vi "YKMW100 Get Com Log.vi"(0 "VISA session":refnum<visa-resource-name>="MW100", 2 "Semiphore":T1, 9 "Timeout (25000)":u32=100, 11 "error in (no error)":errorcluster, 13 "Source (\"\")":string) -> (4 "dup VISA session":refnum<visa-resource-name>, 6 "Com History":string[](array[string]), 7 "Send Message (\"\")":string, 15 "error out":errorcluster)   [LabVIEW 2009]
doc: "This VI sends the message. Then it returns the response."
panel:
  out "Read Buffer":string
  in  "Number of Read Blocks (1-200)":i32=200
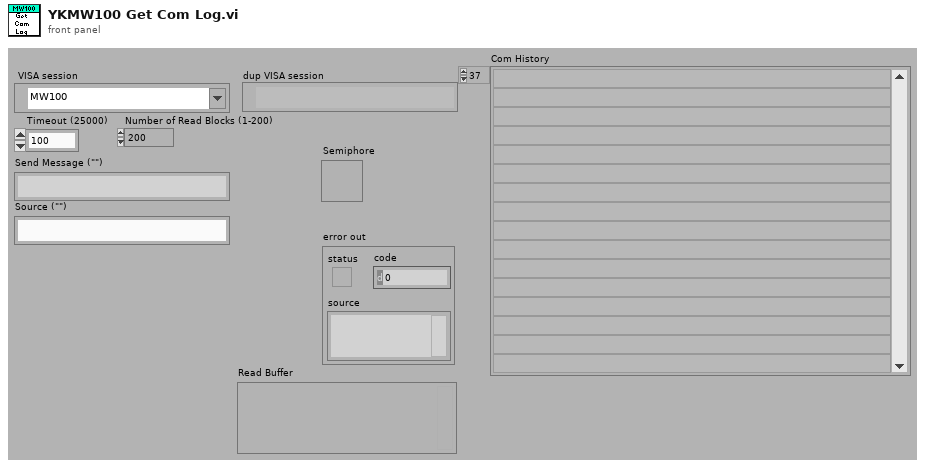
[diagram p1: front panel]
types:
  T1 = typedef "Semaphore RefNum" = refnum<k1>
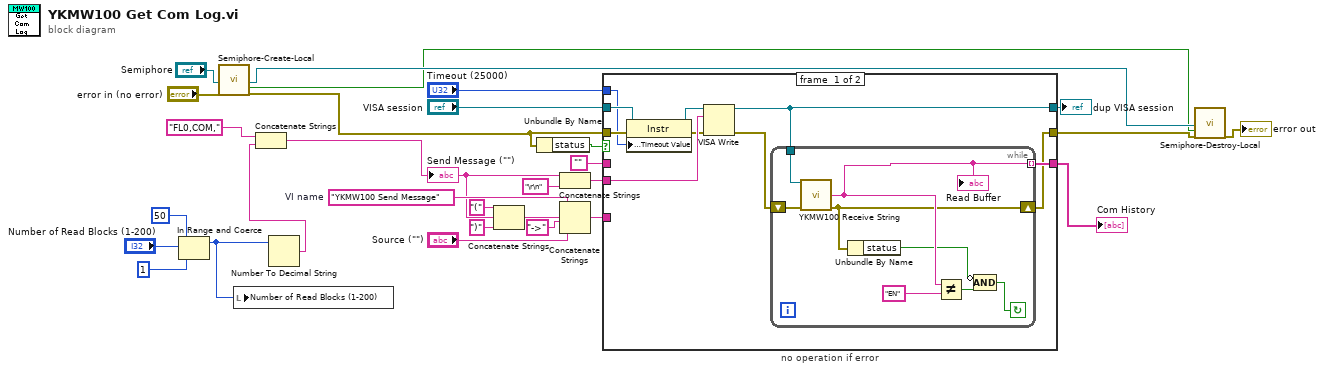
[diagram p0: block diagram]
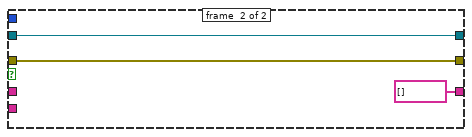
[diagram p2: hidden frame]
diagram:
  w19 = "YKMW100 Send Message"  # VI name
  n1 = In Range and Coerce(upper limit=50, x="Number of Read Blocks (1-200)", lower limit=1) -> (coerced(x)=w11:i32)  [unwired: 1 out]
  n2 = call "Semiphore-Create-Local.vi"("Semiphore"="Semiphore", "error in (no error)"="error in (no error)") -> ("semaphore"=w2:T1, "Local?"=w1:bool, "error out"=w5:errorcluster)  [unwired: 15 in]
  n3 = local write "Number of Read Blocks (1-200)"(w11) -> ()
  n4 = Number To Decimal String(number=w11) -> (decimal integer string=w10:string)  [unwired: 1 in]
  n5 = Concatenate Strings("FL0,COM,", w10) -> (w9:string)
  "Send Message (\"\")" <- w9
  n6 = Concatenate Strings("(", w9, ")") -> (w20:string)
  n7 = Unbundle By Name(w5) -> ("status"=w26:bool)
  n8 = Concatenate Strings(w9, "\r\n") -> (w29:string)
  n9 = Concatenate Strings(w19, w20, "->", "Source (\"\")") -> (w25:string)
  n10 = case "no operation if error" shown="False" w26 {
    tunnel: "VISA session" -> [w36 w50]
    tunnel: w29 -> [w39 _]
    tunnel: [w30 w50] -> w18
    tunnel: [w32 w49] -> w4
    tunnel: w5 -> [w38 w49]
    tunnel: w25 -> [_ _]
    tunnel: "Timeout (25000)" -> [w34 _]
    tunnel: [w33 string[] []] -> w8
    tunnel: "" -> [_ _]
    frame #0 {
      n11 = property class="Instr"(reference=w36, error in=w38, "General Settings:Timeout Value"=w34) -> (reference out=w35:refnum<visa-resource-name>, error out=w37:errorcluster)
      n12 = VISA Write(VISA resource name=w35, write buffer=w39, error in (no error)=w37) -> (VISA resource name out=w30:refnum<visa-resource-name>, error out=w31:errorcluster)  [unwired: 1 out]
      n13 = while {
        tunnel: w30 -> [w47]
        tunnel: [w45] -> w33 mode=indexing
        shift-right: [w41] -> w32
        shift-left: w31 -> [w46]
        stop <- w42 continue-if-true
        n14 = call "YKMW100 Receive String.vi"("VISA session"=w47, "error in (no error)"=w46) -> ("Read Buffer"=w45:string, "error out"=w41:errorcluster)  [unwired: 11 in, 1 out]
        "Read Buffer" <- w45
        n15 = Unbundle By Name(w41) -> ("status"=w43:bool)
        n16 = Not Equal?(x=w45, y="EN" ("concatenated string")) -> (x != y?=w44:bool)
        n17 = Compound Arithmetic op=AND(invert w43, w44) -> (w42:bool)
      }
    }
    frame #1 {
    }
  }
  "dup VISA session" <- w18
  "Com History" <- w8
  n18 = call "Semiphore-Destroy-Local.vi"("Semiphore"=w2, "Local?"=w1, "error in (no error)"=w4) -> ("error out"=→"error out":errorcluster)  [unwired: 16 in]
